vi "adjustAngle_02.vi"() -> ()   [LabVIEW 2011]
panel:
  in  "Move to ref angle first":bool=TRUE
  in  "time done (s)":dbl
  in  "time to wait (s)":dbl=2.0
  out "Wait to set":bool
  in  "Ref Angle (deg)":dbl=30.0 format="%.1f"
  out "IO error":errorcluster
  in  "stop":bool
  out "Angle Indicator (deg)":dbl=20.6 caption="Angle (deg)" format="%.1f"
  in  "Angle (deg)":dbl format="%.1f"
  out "P (torr)":dbl=19.959999999999997 format="%.2f"
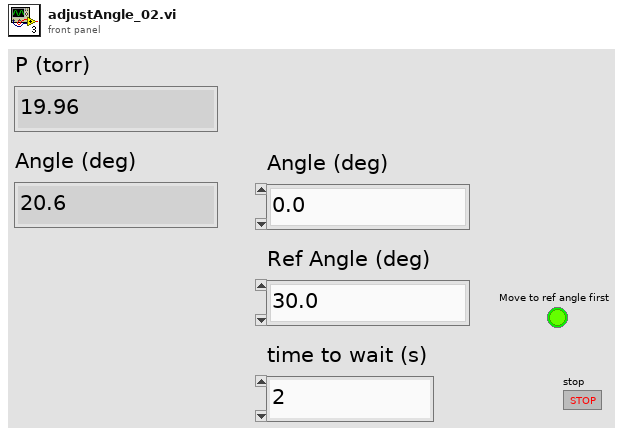
[diagram p1: front panel]
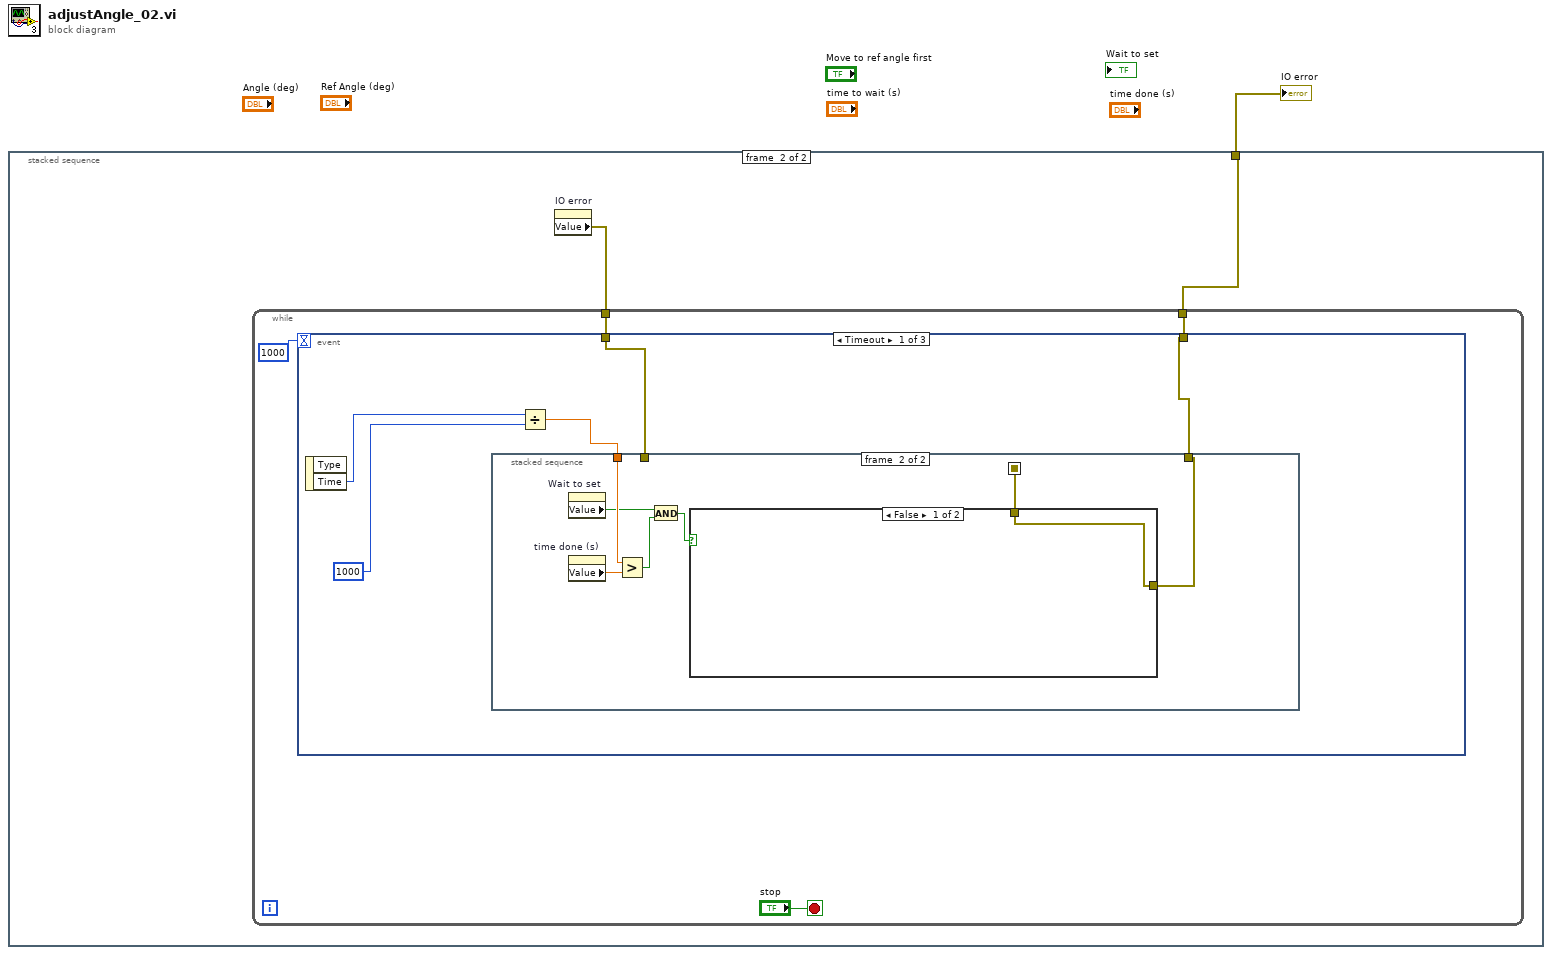
[diagram p0: block diagram]
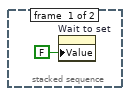
[diagram p2: hidden frame]
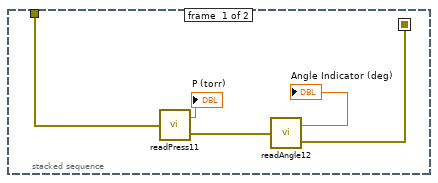
[diagram p3: hidden frame]
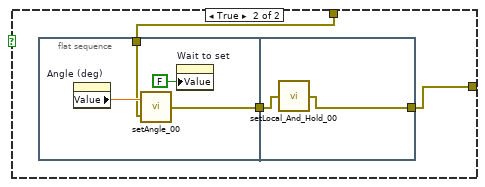
[diagram p4: hidden frame]
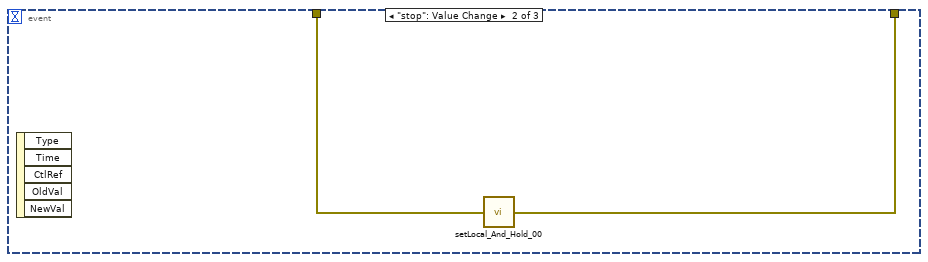
[diagram p5: hidden frame]
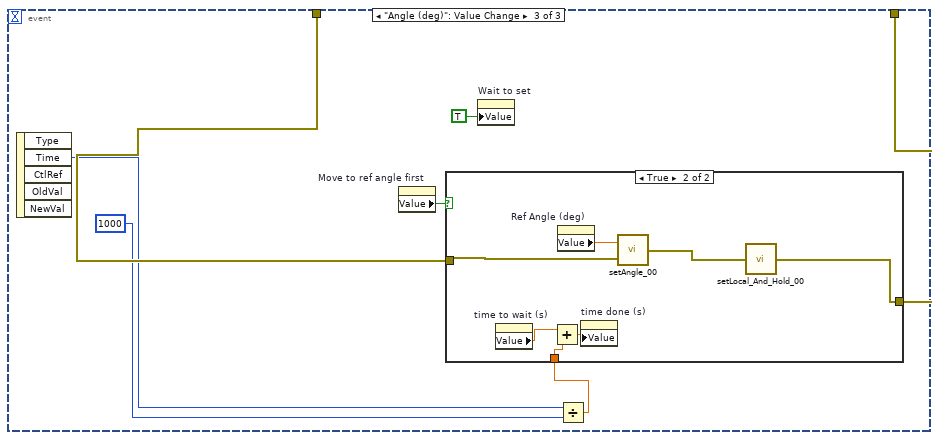
[diagram p6: hidden frame]
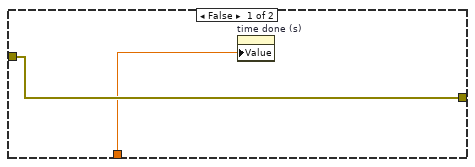
[diagram p7: hidden frame]
diagram:
  n1 = stacked-sequence {
    tunnel: [_ w3] -> w1
    frame #0 {
      n2 = property on="Wait to set" class="Bool (strict)"("Value"=FALSE ("Wait to set")) -> ()  [unwired: 2 in, 2 out]
    }
    frame #1 {
      n3 = property on="IO error" class="Clust (strict)"() -> ("Value"=w4:errorcluster)  [unwired: 2 in, 2 out]
      n4 = while {
        tunnel: w4 -> [w7]
        tunnel: [w6] -> w3
        stop <- "stop" stop-if-true
        n5 = event shown="[0] Timeout" {
          selector: _ -> [_ _ _]
          dyn-events: _ -> [_ _ _]
          timeout: 1000 -> [_ _ _]
          tunnel: w7 -> [w13 w37 w43]
          tunnel: [w12 w36 w44] -> w6
          event Timeout {
            n6 = event-data() -> ("Time"=w11:u32)  [unwired: 1 in, 1 out]
            n7 = Divide(x=w11, y=u32 1000) -> (x/y=w9:dbl)
            n8 = stacked-sequence {
              seq-local: [w14 _] -> [_ w19]
              tunnel: w13 -> [w18 _]
              tunnel: w9 -> [_ w25]
              tunnel: [_ w21] -> w12
              frame #0 {
                n9 = call "readPress11.vi"("error in"=w18) -> ("P"=→"P (torr)":dbl, "error out"=w15:errorcluster)
                n10 = call "readAngle12.vi"("error in"=w15) -> ("angle"=→"Angle Indicator (deg)":dbl, "error out"=w14:errorcluster)
              }
              frame #1 {
                n11 = property on="Wait to set" class="Bool (strict)"() -> ("Value"=w20:bool)  [unwired: 2 in, 2 out]
                n12 = property on="time done (s)" class="DigNum (strict)"() -> ("Value"=w24:dbl)  [unwired: 2 in, 2 out]
                n13 = Greater?(x=w25, y=w24) -> (0:w23:bool)
                n14 = And(x=w20, y=w23) -> (x .and. y?=w22:bool)
                n15 = case shown="False" w22 {
                  tunnel: [w26 w29] -> w21
                  tunnel: w19 -> [w26 w27]
                  frame False {
                  }
                  frame True {
                    n16 = flat-sequence {
                      tunnel: [w32] -> w28
                      tunnel: w27 -> [w30]
                      tunnel: [w34] -> w29
                      tunnel: w28 -> [w35]
                      frame #0 {
                        n17 = property on="Angle (deg)" class="DigNum (strict)"() -> ("Value"=w33:dbl)  [unwired: 2 in, 2 out]
                        n18 = call "setAngle_00.vi"("error in (no error)"=w30, "Angle (deg)"=w33) -> ("error out"=w32:errorcluster)
                        n19 = property on="Wait to set" class="Bool (strict)"("Value"=FALSE ("Wait to set")) -> ()  [unwired: 2 in, 2 out]
                      }
                      frame #1 {
                        n20 = call "setLocal_And_Hold_00.vi"("error in (no error)"=w35) -> ("error out"=w34:errorcluster)
                      }
                    }
                  }
                }
              }
            }
          }
          event "stop": Value Change {
            n21 = event-data() -> ()  [unwired: 1 in, 5 out]
            n22 = call "setLocal_And_Hold_00.vi"("error in (no error)"=w37) -> ("error out"=w36:errorcluster)
          }
          event "Angle (deg)": Value Change {
            n23 = event-data() -> ("Time"=w42:u32)  [unwired: 1 in, 4 out]
            n24 = property on="Move to ref angle first" class="Bool (strict)"() -> ("Value"=w39:bool)  [unwired: 2 in, 2 out]
            n25 = property on="Wait to set" class="Bool (strict)"("Value"=TRUE ("Wait to set")) -> ()  [unwired: 2 in, 2 out]
            n26 = Divide(x=w42, y=u32 1000) -> (x/y=w40:dbl)
            n27 = case shown="True" w39 {
              tunnel: w43 -> [w46 w52]
              tunnel: [w46 w47] -> w44
              tunnel: w40 -> [w45 w49]
              frame False {
                n28 = property on="time done (s)" class="DigNum (strict)"("Value"=w45) -> ()  [unwired: 2 in, 2 out]
              }
              frame True {
                n29 = property on="time to wait (s)" class="DigNum (strict)"() -> ("Value"=w50:dbl)  [unwired: 2 in, 2 out]
                n30 = Add(x=w50, y=w49) -> (x+y=w51:dbl)
                n31 = property on="Ref Angle (deg)" class="DigNum (strict)"() -> ("Value"=w53:dbl)  [unwired: 2 in, 2 out]
                n32 = property on="time done (s)" class="DigNum (strict)"("Value"=w51) -> ()  [unwired: 2 in, 2 out]
                n33 = call "setAngle_00.vi"("error in (no error)"=w52, "Angle (deg)"=w53) -> ("error out"=w48:errorcluster)
                n34 = call "setLocal_And_Hold_00.vi"("error in (no error)"=w48) -> ("error out"=w47:errorcluster)
              }
            }
          }
        }
      }
    }
  }
  "IO error" <- w1
